vi "main1.vi"() -> ()   [LabVIEW 2022 SP3]
uses:
  Control 1.ctl
  <vilib>/numeric/Random Number (Range) DBL.vi
panel:
  out "String":string
  out "x = y?":bool
  out "x .and. y?":bool
  in  "Symulowana_godzina":string="This is a text.\nHere is a new line.\n\nAnd that's another."
  out "Godziny_jako_array":string[](array[string])
  in  "Godziny_otwarcia":string="8:00\n8:30\n9:00\n9:30\n10:00\n10:30\n11:00\n11:30\n12:00\n12:30\n13:00\n13:30\n14:00\n14:30\n15:00\n15:30\n16:00\n16:30\n17:00\n17:30\n18:00\n18:30\n19:00\n19:30"
  out "Obecna godzina":string
  out "Data i godzina":timestamp
  in  "Start sluza proces 2":bool
  out "Niski    ----> Wysoki":bool
  out "Wysoki ----> Niski":bool
  in  "Zalaczenie sluzy":bool
  out "Wrota zamkniete":bool
  in  "Stopien zamkniecia wrot 2":dbl(slide) scale=0.0..10.0
  in  "Poziom zamkniecia wrot 1":dbl(slide) scale=0.0..10.0
  in  "Start sluza proces":bool
  in  "stop":bool
  out "Poziom wody za sluza":dbl(slide)=8.064516129032258 scale=0.0..10.0
  out "Poziom wody w sluzie":dbl(slide)=4.0 scale=0.0..10.0
  out "Poziom wody przed sluza":dbl(slide)=4.129032258064516 scale=0.0..10.0
  # "Kamera 1"
  # "Kamera 2"
  # "Nastepny kierunkek sluzy:"
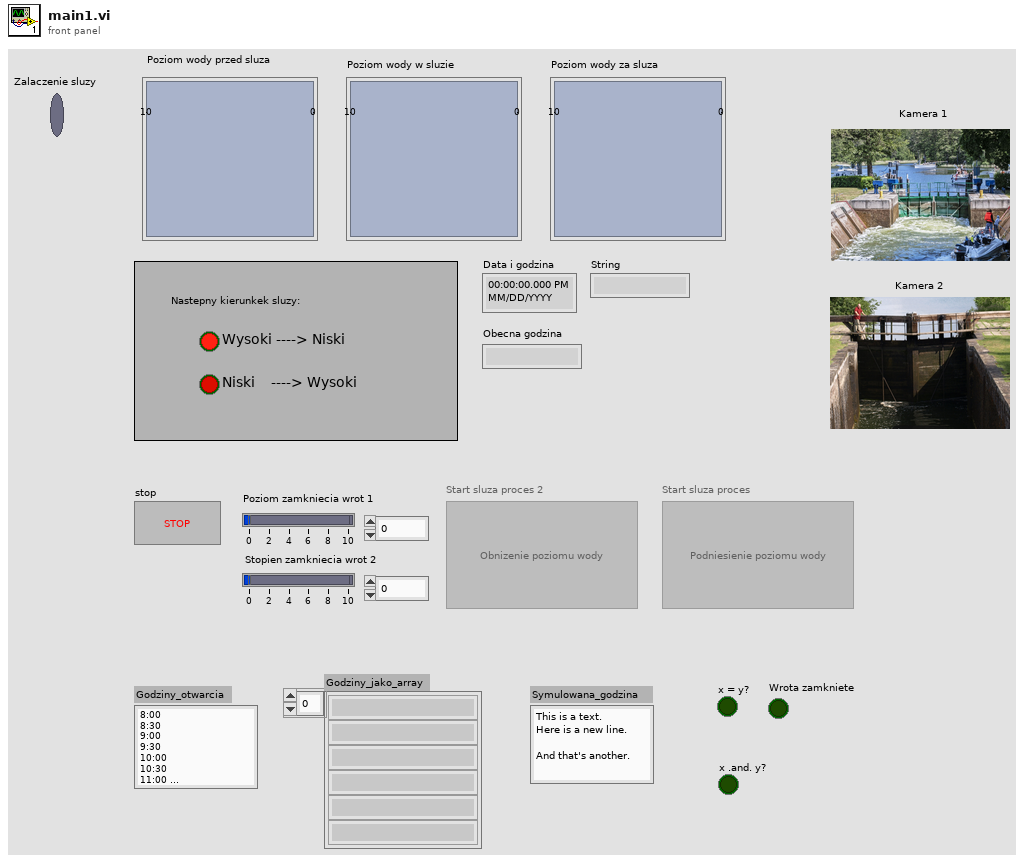
[diagram p1: front panel]
types:
  T1 = typedef "Control 1.ctl" = enum16{"Init", "Idle", "Monitor", "Process_2", "Process", "Exit"}
  T2 = enum8{"Enabled", "Disabled", "Disabled and Grayed Out"}
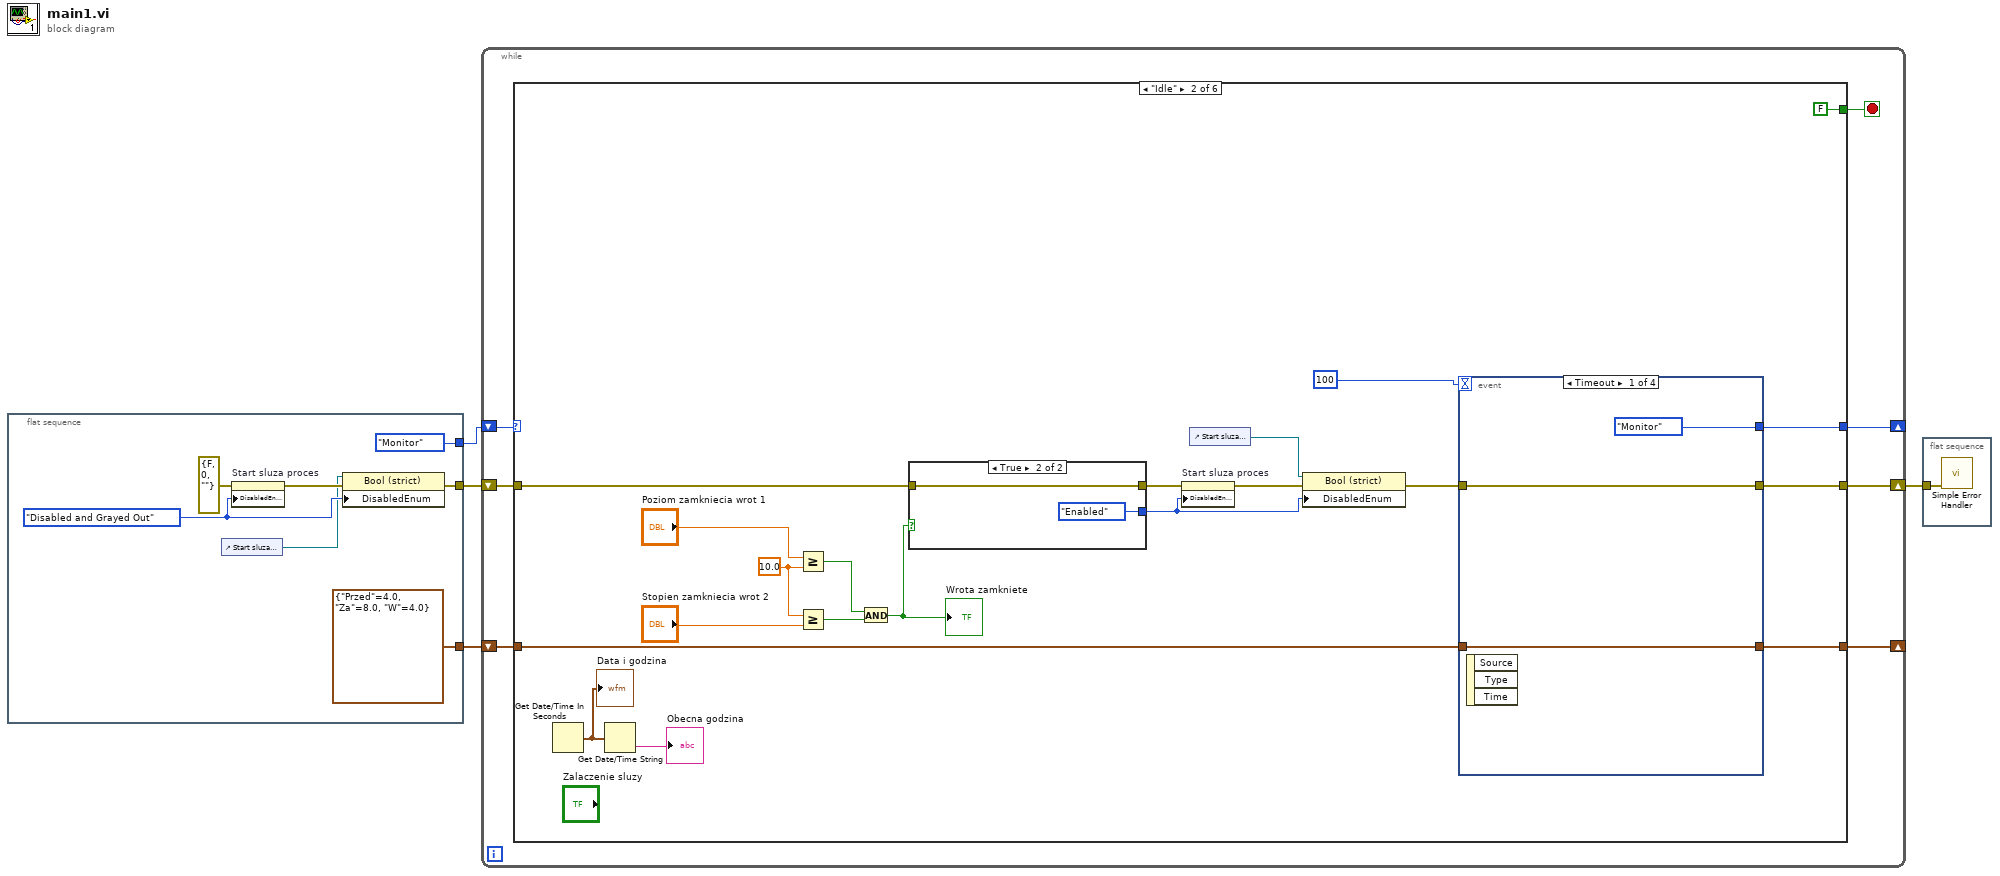
[diagram p0: block diagram]
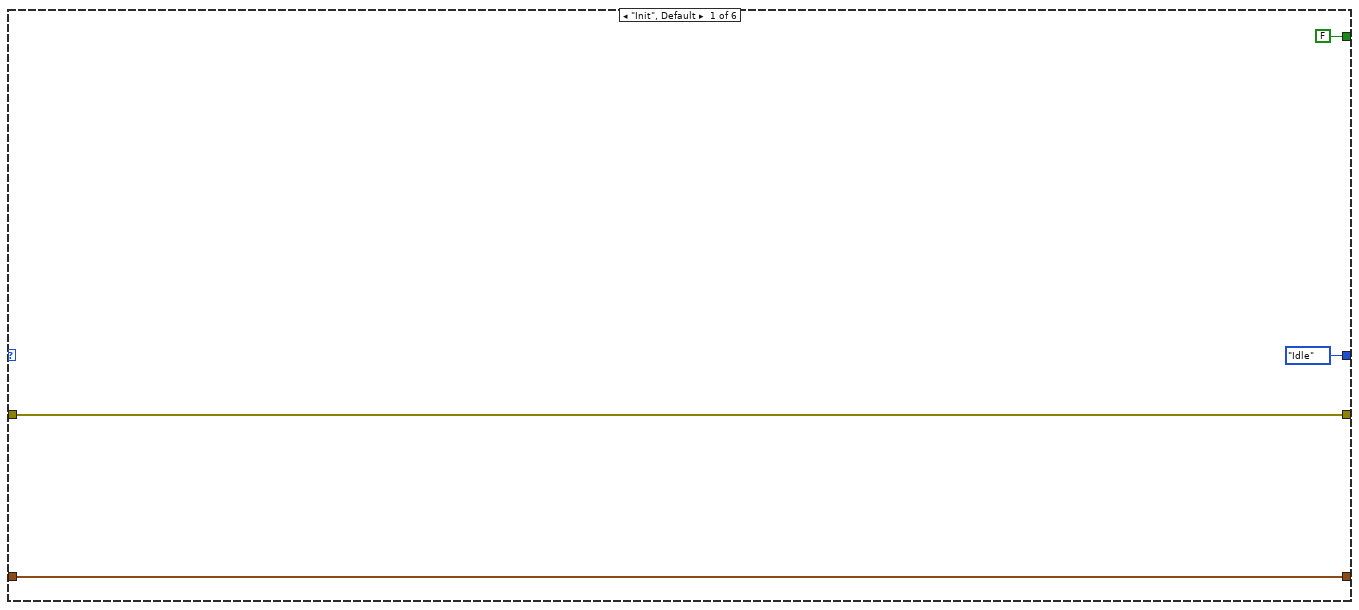
[diagram p2: hidden frame]
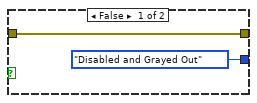
[diagram p3: hidden frame]
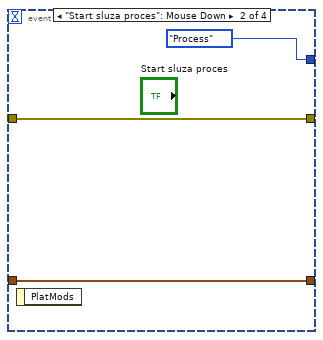
[diagram p4: hidden frame]
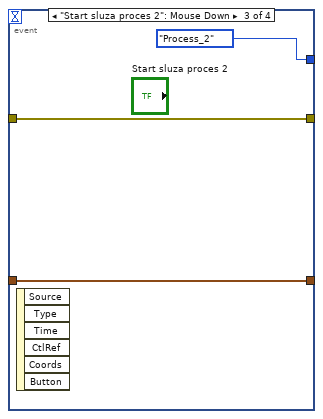
[diagram p5: hidden frame]
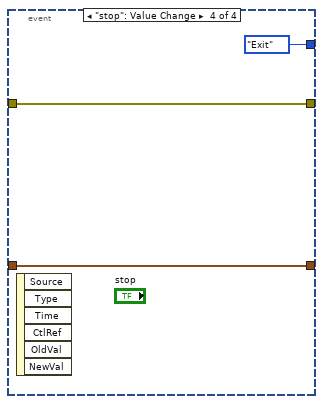
[diagram p6: hidden frame]
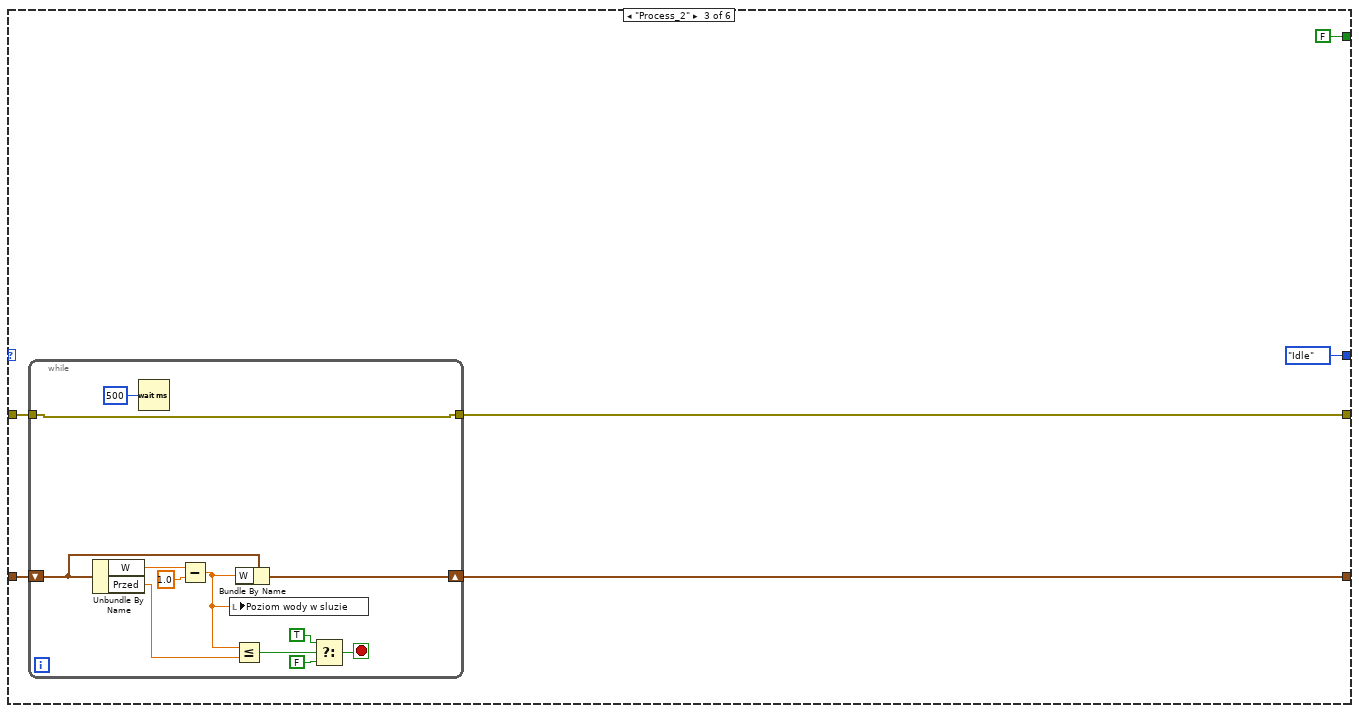
[diagram p7: hidden frame]
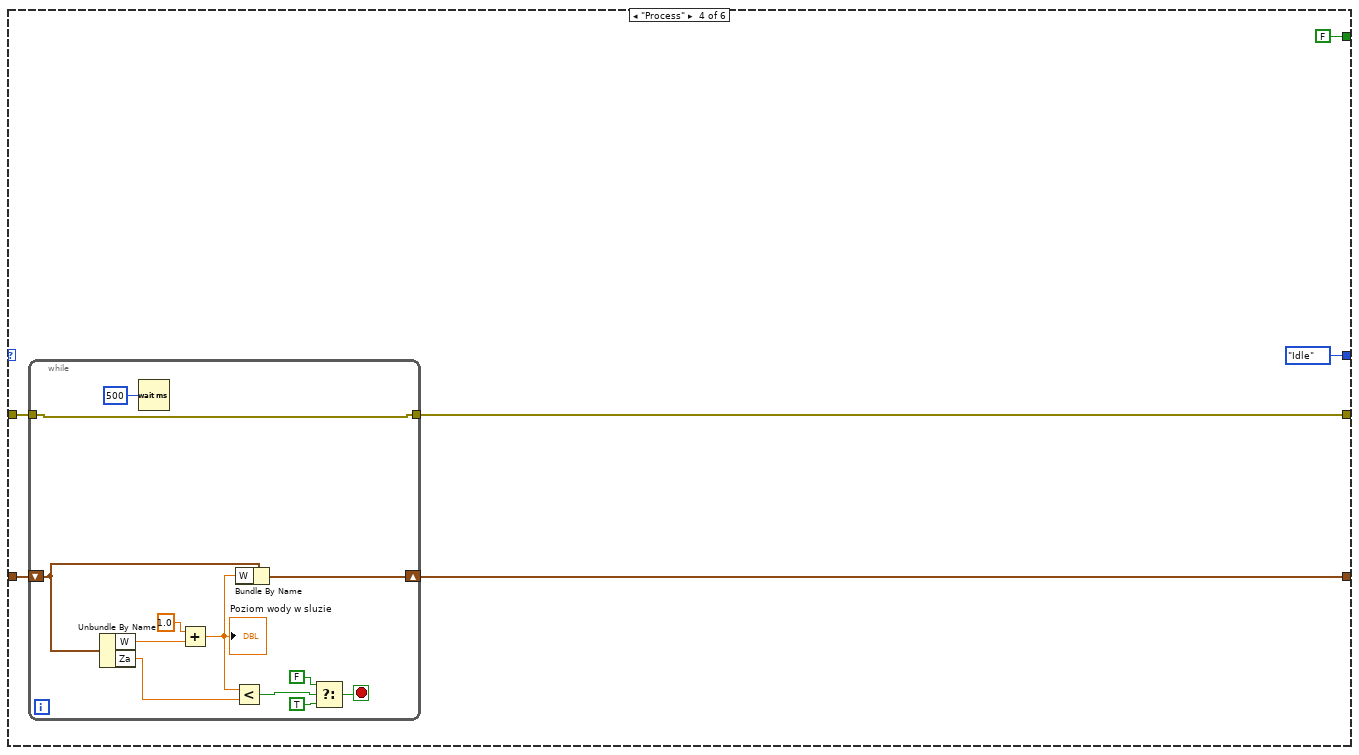
[diagram p8: hidden frame]
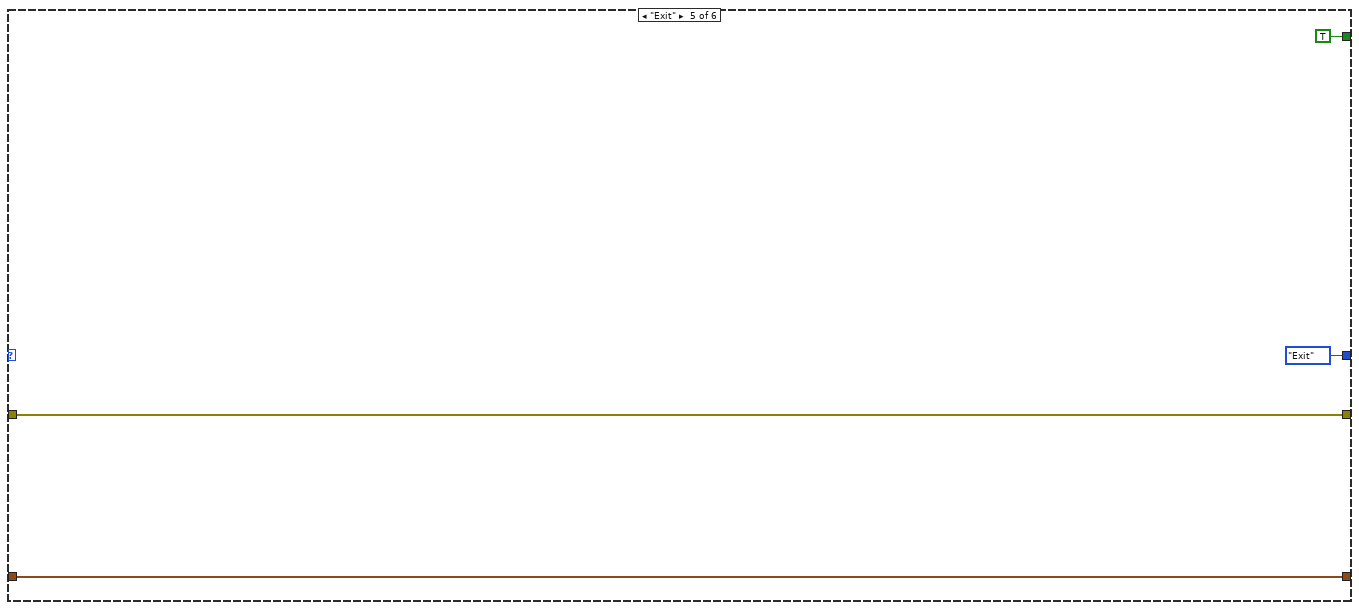
[diagram p9: hidden frame]
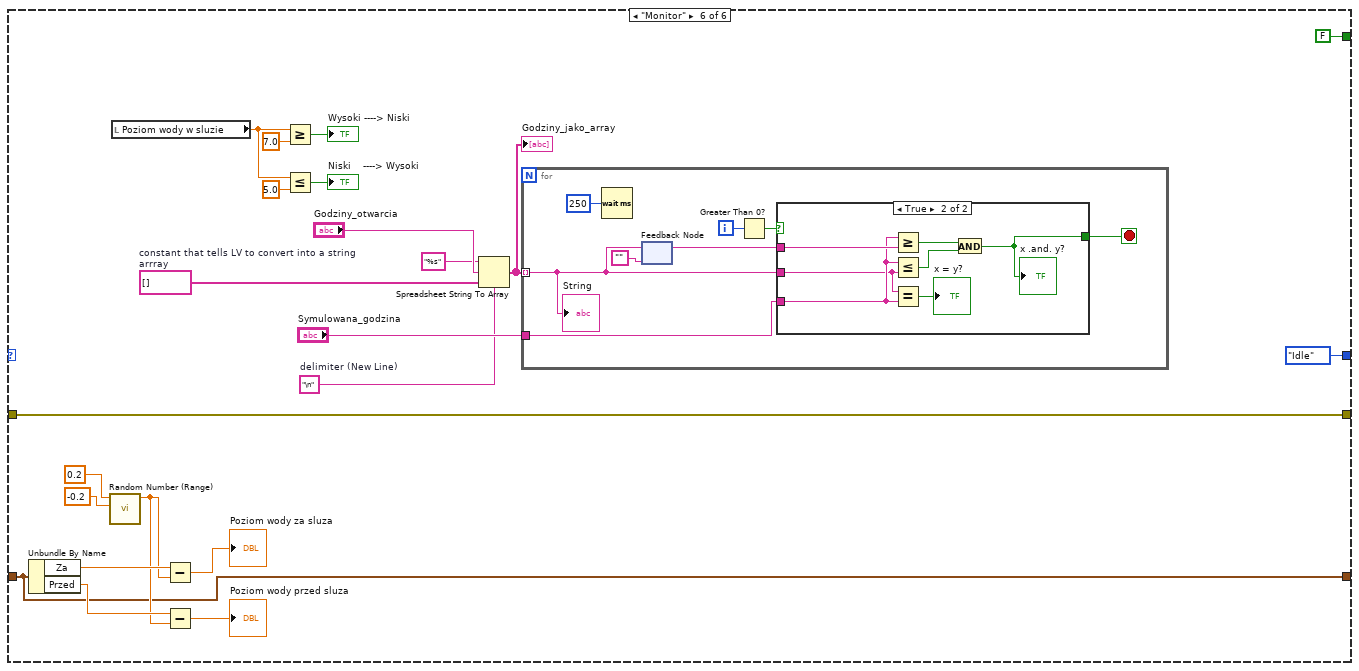
[diagram p10: hidden frame]
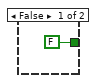
[diagram p11: hidden frame]
diagram:
  n1 = flat-sequence {
    tunnel: [cluster{"Przed":dbl, "Za":dbl, "W":dbl} {"Przed"=4.0, "Za"=8.0, "W"=4.0}] -> w4
    tunnel: [Control_1."Monitor"] -> w3
    tunnel: [w5] -> w2
    frame #0 {
      w7 = T2."Disabled and Grayed Out" ("Disabled")
      n2 = control-ref of="Start sluza proces 2"() -> (w6:refnum<vi>)
      n3 = property on="Start sluza proces" class="Bool (strict)"(error in=errorcluster {"status"=FALSE, "code"=0, "source"=""} ("error constant"), "DisabledEnum"=w7) -> (error out=w8:errorcluster)  [unwired: 1 in, 1 out]
      n4 = property on="Property Node" class="Bool (strict)"(reference=w6, error in=w8, "DisabledEnum"=w7) -> (error out=w5:errorcluster)  [unwired: 1 out]
    }
  }
  n5 = while {
    shift-right: [w13] -> w1
    shift-left: w2 -> [w12]
    shift-right: [w17] -> _
    shift-left: w4 -> [w16]
    shift-right: [w15] -> _
    shift-left: w3 -> [w18]
    stop <- w14 stop-if-true
    n6 = case shown="\"Idle\"" w18 {
      tunnel: [w19 w40 w62 w80 w96 w113] -> w17
      tunnel: w16 -> [w19 w39 w63 w77 w96 w113]
      tunnel: [Control_1."Idle" w41 Control_1."Idle" Control_1."Idle" Control_1."Exit" Control_1."Idle"] -> w15
      tunnel: [FALSE FALSE FALSE FALSE TRUE FALSE] -> w14
      tunnel: [w20 w38 w60 w79 w95 w114] -> w13
      tunnel: w12 -> [w20 w32 w61 w78 w95 w114]
      frame "Init", Default {
      }
      frame "Idle" {
        w33 = 10.0
        n7 = Get Date/Time In Seconds() -> (seconds since 1Jan1904=w25:timestamp)
        "Data i godzina" <- w25
        n8 = Get Date/Time String(seconds (now)=w25) -> (time string=→"Obecna godzina":string)  [unwired: 2 in, 1 out]
        n9 = Greater Or Equal?(x="Poziom zamkniecia wrot 1", y=w33) -> (x >= y?=w36:bool)
        n10 = Greater Or Equal?(x=w33, y="Stopien zamkniecia wrot 2") -> (x >= y?=w35:bool)
        n11 = And(x=w36, y=w35) -> (x .and. y?=w31:bool)
        "Wrota zamkniete" <- w31
        n12 = case shown="True" w31 {
          tunnel: w32 -> [w44 w45]
          tunnel: [w44 w45] -> w30
          tunnel: [T2."Disabled and Grayed Out" ("Disabled") T2."Enabled" ("Disabled")] -> w27
          frame False {
          }
          frame True {
          }
        }
        n13 = property on="Start sluza proces" class="Bool (strict)"(error in=w30, "DisabledEnum"=w27) -> (error out=w29:errorcluster)  [unwired: 1 in, 1 out]
        n14 = control-ref of="Start sluza proces 2"() -> (w26:refnum<vi>)
        n15 = property on="Property Node" class="Bool (strict)"(reference=w26, error in=w29, "DisabledEnum"=w27) -> (error out=w28:errorcluster)  [unwired: 1 out]
        n16 = event shown="[0] Timeout" {
          selector: _ -> [_ _ _ _]
          dyn-events: _ -> [_ _ _ _]
          timeout: 100 -> [_ _ _ _]
          tunnel: [Control_1."Monitor" Control_1."Process" Control_1."Process_2" Control_1."Exit"] -> w41
          tunnel: [w48 w51 w54 w58] -> w40
          tunnel: w39 -> [w48 w51 w54 w58]
          tunnel: [w47 w50 w55 w56] -> w38
          tunnel: w28 -> [w47 w50 w55 w56]
          event Timeout {
            n17 = event-data() -> ()  [unwired: 1 in, 3 out]
          }
          event "Start sluza proces": Mouse Down {
            n18 = event-data() -> ()  [unwired: 1 in, 1 out]
          }
          event "Start sluza proces 2": Mouse Down {
            n19 = event-data() -> ()  [unwired: 1 in, 6 out]
          }
          event "stop": Value Change {
            n20 = event-data() -> ()  [unwired: 1 in, 6 out]
          }
        }
      }
      frame "Process_2" {
        n21 = while {
          shift-right: [w68] -> w62
          shift-left: w63 -> [w70]
          tunnel: w61 -> [w65]
          tunnel: [w65] -> w60
          stop <- w71 stop-if-true
          n22 = Unbundle By Name(w70) -> ("W"=w76:dbl, "Przed"=w66:dbl)
          n23 = Wait (ms)(milliseconds to wait=u32 500) -> ()  [unwired: 1 out]
          n24 = Subtract(x=w76, y=1.0) -> (x-y=w69:dbl)
          n25 = local write "Poziom wody w sluzie"(w69) -> ()
          n26 = Less Or Equal?(x=w69, y=w66) -> (x <= y?=w74:bool)
          n27 = Bundle By Name(cluster=w70, "W"=w69) -> (w68:cluster{"Przed":dbl, "Za":dbl, "W":dbl})
          n28 = Select(t=TRUE, s=w74, f=FALSE) -> (s? t:f=w71:bool)
        }
      }
      frame "Process" {
        n29 = while {
          shift-right: [w91] -> w80
          shift-left: w77 -> [w90]
          tunnel: [w85] -> w79
          tunnel: w78 -> [w85]
          stop <- w88 stop-if-true
          n30 = Unbundle By Name(w90) -> ("W"=w83:dbl, "Za"=w84:dbl)
          n31 = Wait (ms)(milliseconds to wait=u32 500) -> ()  [unwired: 1 out]
          n32 = Add(x=1.0, y=w83) -> (x+y=w86:dbl)
          "Poziom wody w sluzie" <- w86
          n33 = Less?(x=w86, y=w84) -> (x < y?=w94:bool)
          n34 = Bundle By Name(cluster=w90, "W"=w86) -> (w91:cluster{"Przed":dbl, "Za":dbl, "W":dbl})
          n35 = Select(t=FALSE, s=w94, f=TRUE) -> (s? t:f=w88:bool)
        }
      }
      frame "Exit" {
      }
      frame "Monitor" {
        w103 = "\n"  # delimiter (New Line)
        w102 = string[] []  # constant that tells LV to convert into a string arrray
        n36 = Unbundle By Name(w113) -> ("Za"=w116:dbl, "Przed"=w117:dbl)
        n37 = call-poly <vilib>:"Random Number (Range).vi"("lower bound (0)"=-0.2, "upper bound (100)"=0.2) -> ("number"=w115:dbl)  [unwired: 9 in]
        n38 = local read "Poziom wody w sluzie"() -> (w109:dbl)
        n39 = Subtract(x=w116, y=w115) -> (x-y=→"Poziom wody za sluza":dbl)
        n40 = Subtract(x=w117, y=w115) -> (x-y=→"Poziom wody przed sluza":dbl)
        n41 = Greater Or Equal?(x=w109, y=7.0) -> (x >= y?=→"Wysoki ----> Niski":bool)
        n42 = Less Or Equal?(x=w109, y=5.0) -> (x <= y?=→"Niski    ----> Wysoki":bool)
        n43 = Spreadsheet String To Array(delimiter (Tab)=w103, format string="%s", spreadsheet string="Godziny_otwarcia", array type (2D Dbl)=w102) -> (array=w104:string[])
        "Godziny_jako_array" <- w104
        n44 = for {
          tunnel: w104 -> [w123] mode=indexing
          tunnel: "Symulowana_godzina" -> [w128]
          i -> [w124]
          stop <- w127 stop-if-true
          n45 = Wait (ms)(milliseconds to wait=u32 250 ("millisecond timer value")) -> ()  [unwired: 1 out]
          n46 = feedback-in #1(w123) -> ()
          n47 = feedback #1("") -> (w121:string)
          n48 = Greater Than 0?(x=w124) -> (x > 0?=w125:bool)
          n49 = case shown="True" w125 {
            tunnel: w123 -> [_ w133]
            tunnel: w128 -> [_ w134]
            tunnel: [FALSE w130] -> w127
            tunnel: w121 -> [_ w135]
            frame False {
            }
            frame True {
              n50 = Greater Or Equal?(x=w134, y=w135) -> (x >= y?=w131:bool)
              n51 = Less Or Equal?(x=w134, y=w133) -> (x <= y?=w132:bool)
              n52 = Equal?(x=w133, y=w134) -> (x = y?=→"x = y?":bool)
              n53 = And(x=w131, y=w132) -> (x .and. y?=w130:bool)
              "x .and. y?" <- w130
            }
          }
          "String" <- w123
        }
      }
    }
  }
  n54 = flat-sequence {
    tunnel: w1 -> [w137]
    frame #0 {
      n55 = call <vilib>:"Simple Error Handler.vi"("error in (no error)"=w137) -> ()  [unwired: 4 in, 5 out]
    }
  }
